vi "DSF.Memory.Buffer.Config.Read.0D.Channel Size.vi"(8 "error in (no error)":errorcluster, 10 "channel index":u64, 11 "Buffer Config in":refnum<class "DSF.Memory.Buffer.Config.lvclass">) -> (0 "error out":errorcluster, 1 "size":u64, 3 "Buffer Config out":refnum<class "DSF.Memory.Buffer.Config.lvclass">)   [LabVIEW 2016, in "DSF.Memory.Buffer.Config.lvclass"]
uses:
  DSF.Memory.Buffer.Config.lvclass
  Memory.Pointer/DSF.Memory.Pointer.U64.lvclass
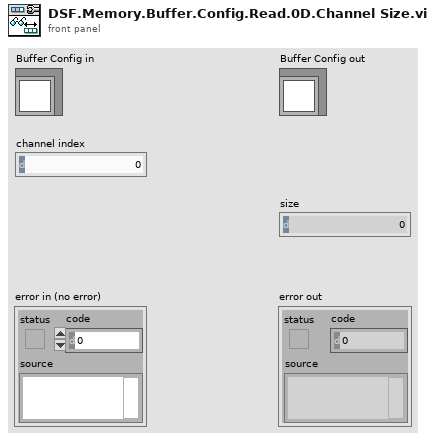
[diagram p1: front panel]
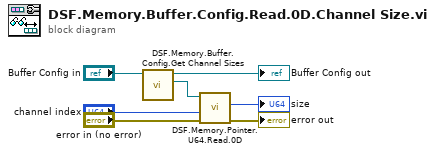
[diagram p0: block diagram]
diagram:
  n1 = call "DSF.Memory.Buffer.Config.Get Channel Sizes.vi"("Buffer Config in"="Buffer Config in") -> ("channel sizes ptr"=w5:refnum<class "DSF.Memory.Pointer.U64.lvclass">, "Buffer Config out"=→"Buffer Config out":refnum<class "DSF.Memory.Buffer.Config.lvclass">)  [unwired: 8 in, 1 out]
  n2 = call "DSF.Memory.Pointer.U64.Read.0D.vi"("error in (no error)"="error in (no error)", "offset (0)"="channel index", "pointer in"=w5) -> ("error out"=→"error out":errorcluster, "value out"=→"size":u64)  [unwired: 5 in, 2 out]
